vi "Teleop.vi"(10 "Match Info":T1={"Autonomous Elapsed Seconds"=0.0, "TeleOp Elapsed Seconds"=0.0, "Disabled Elapsed Seconds"=0.0, "Visited Autonomous"=FALSE, "Visited TeleOp"=FALSE, "Visited Disabled"=FALSE, "Autonomous Settings"={"Autonomous Style"=enum."Independent", "VI Refnum"=refnum}}, 11 "Call Context":T2) -> ()   [LabVIEW 2012]
doc: "This VI is called for each TeleOp packet received from the DS where the robot is not disabled. It is often used to read from the joysticks and update I/O or to update setpoints for timed control loops. It should complete and return within 20 milliseconds or it may miss DS packets."
uses:
  <vilib>/Rock Robotics/WPI/DriverStation/WPI_DriverStationDerivedRobotMode.ctl
  <vilib>/Rock Robotics/WPI/DriverStation/WPI_DriverStationMatch Info.ctl
  Robot Global Data.vi
  <vilib>/Rock Robotics/WPI/Joystick/WPI_JoystickGetSetRefNum.vi
  <vilib>/Rock Robotics/WPI/RobotDrive/WPI_RobotDriveGetSetRefNum.vi
  Documents/LabVIEW Data/No Wayne Drive/wayne drive.vi
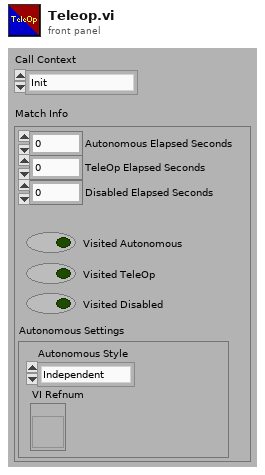
[diagram p1: front panel]
types:
  T1 = typedef "WPI_DriverStationMatch Info.ctl" = cluster{"Autonomous Elapsed Seconds":dbl, "TeleOp Elapsed Seconds":dbl, "Disabled Elapsed Seconds":dbl, "Visited Autonomous":bool, "Visited TeleOp":bool, "Visited Disabled":bool, "Autonomous Settings":cluster{"Autonomous Style":enum16{"Iterative", "Independent"}, "VI Refnum":refnum<vi>}}
  T2 = typedef "WPI_DriverStationDerivedRobotMode.ctl" = enum16{"Init", "Execute", "Stop"}
  T3 = typedef "WPI_JoystickDevRef.ctl" = cluster{"Device":T4}
  T4 = typedef "WPI_JoystickDeviceEnum.ctl" = enum16{"USB 1", "USB 2", "USB 3", "USB 4", "Kinect 1", "Kinect 2"}
  T5 = typedef "WPI_JoystickButtonState.ctl" = cluster{"Button 1":bool, "Button 2":bool, "Button 3":bool, "Button 4":bool, "Button 5":bool, "Button 6":bool, "Button 7":bool, "Button 8":bool, "Button 9":bool, "Button 10":bool, "Button 11":bool, "Button 12":bool}
  T6 = cluster{"axis 1 (x)":dbl, "axis 2 (y)":dbl, "axis 3 (throttle)":dbl, "axis 4":dbl, "axis 5":dbl, "axis 6":dbl}
  T7 = typedef "WPI_RobotDriveDevRef.ctl" = cluster{"DevStatus":errorcluster, "Motors[]":T8[], "Square Inputs":bool, "Max Output":dbl, "Isochronous":bool}
  T8 = typedef "WPI_MotorControlDeviceRef.ctl" = cluster{"DeviceStatus":errorcluster, "Type":enum16{"PWM", "CAN"}, "PWM":cluster{"Digital Module":T9, "PWM Channel":T10, "DeadBand":T11}, "CAN":cluster{"Device Number":u8, "Control Mode":T12, "Semaphore":T13, "Max Vout":dbl}, "Invert":bool, "TransformRef":T14, "InvTransformRef":T14}
  T9 = typedef "FPGA_TypedefDigitalModule.ctl" = enum16{"Digital Module 1", "Digital Module 2"}
  T10 = typedef "FPGA_DIOPWMChannel.ctl" = enum8{"PWM 1", "PWM 2", "PWM 3", "PWM 4", "PWM 5", "PWM 6", "PWM 7", "PWM 8", "PWM 9", "PWM 10", "Invalid"}
  T11 = typedef "WPI_PWMDeadband.ctl" = cluster{"Name":string, "maxPositivePwm":i32, "minPositivePwm":i32, "centerPwm":i32, "maxNegativePwm":i32, "minNegativePwm":i32, "angularRange":u16}
  T12 = typedef "WPI_CANJaguar_ControlMode.ctl" = enum8{"Percent VBus", "Current", "Speed", "Position", "Voltage"}
  T13 = typedef "Semaphore RefNum" = refnum<k1>
  T14 = typedef "WPI_PWMTransform_ConPane.ctl" = refnum<vi>
  T15 = typedef "WPI_RelayDevRef.ctl" = cluster{"DevStatus":errorcluster, "Relay Channel":T16, "Digital Module":T9, "Relay Direction":T17}
  T16 = typedef "FPGA_DIORelayChannel.ctl" = enum8{"Relay 1", "Relay 2", "Relay 3", "Relay 4", "Relay 5", "Relay 6", "Relay 7", "Relay 8", "Invalid"}
  T17 = typedef "WPI_RelayDirection.ctl" = enum16{"Both directions", "Forward only", "Reverse only"}
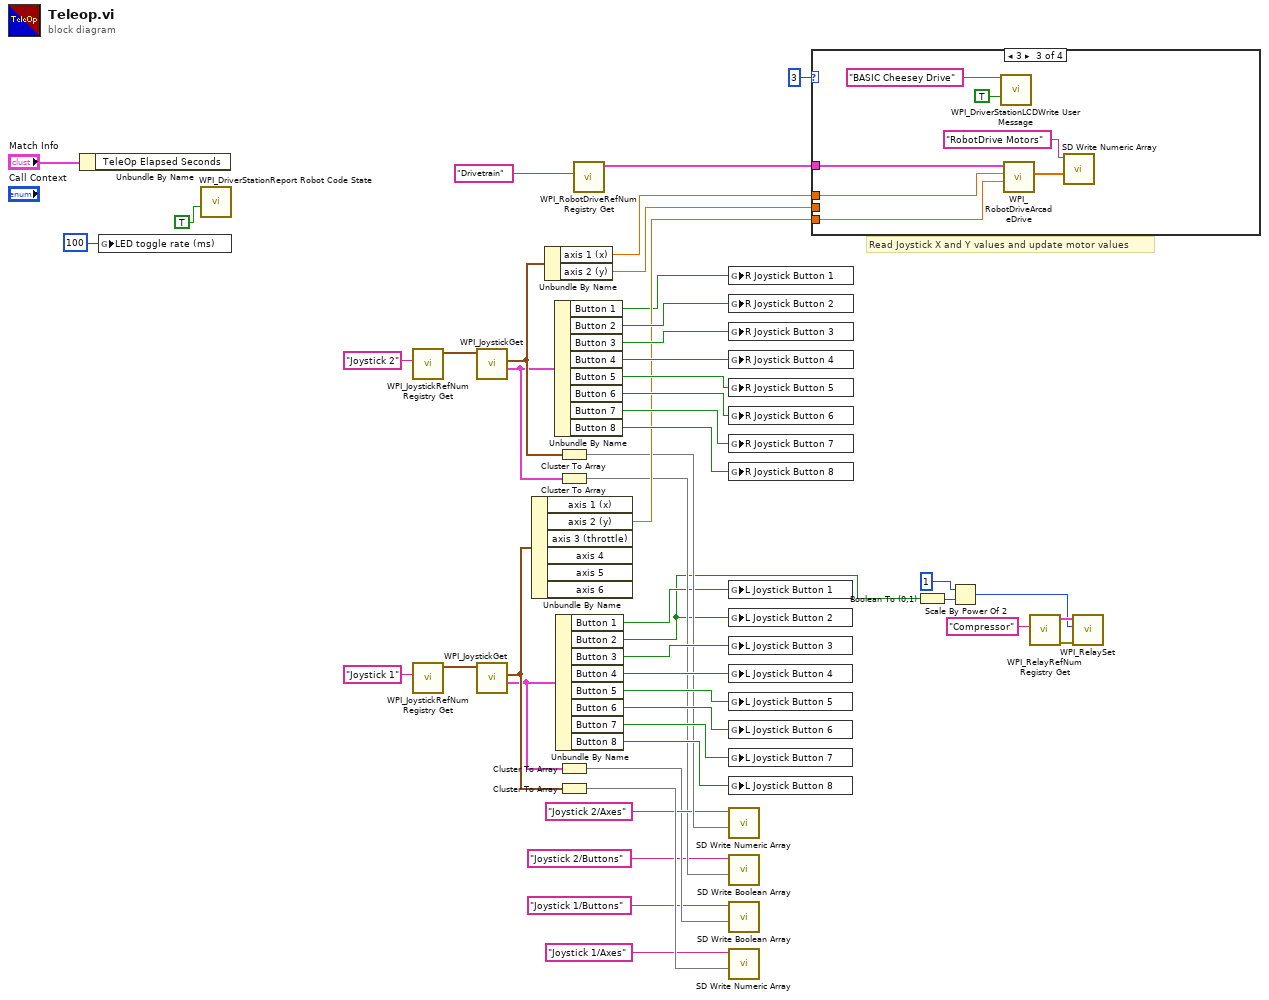
[diagram p0: block diagram]
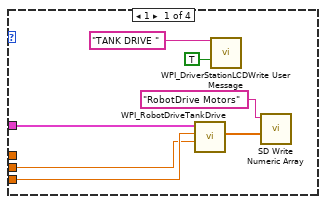
[diagram p2: hidden frame]
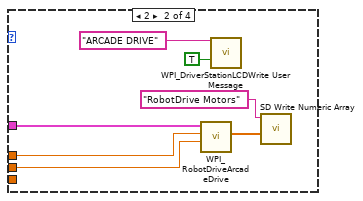
[diagram p3: hidden frame]
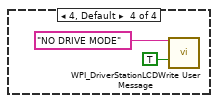
[diagram p4: hidden frame]
diagram:
  # "Read Joystick X and Y values and update motor values"
  n1 = Unbundle By Name("Match Info") -> ()  [unwired: 1 out]
  n2 = global write "Robot Global Data.vi" "LED toggle rate (ms)"(u32 100 ("LED ms toggle rate")) -> ()
  n3 = call <vilib>:"WPI_DriverStationReport Robot Code State.vi"("TeleOp"=TRUE ("Autonomous")) -> ()  [unwired: 10 in, 1 out]
  n4 = call <vilib>:"WPI_JoystickRefNum Registry Get.vi"("refnum name"="Joystick 2") -> ("JoystickDevRef"=w40:T3)  [unwired: 1 in, 9 out]
  n5 = call <vilib>:"WPI_JoystickRefNum Registry Get.vi"("refnum name"="Joystick 1") -> ("JoystickDevRef"=w42:T3)  [unwired: 1 in, 9 out]
  n6 = call <vilib>:"WPI_JoystickGet.vi"("JoystickDevRef"=w40) -> ("Buttons"=w11:T5, "Axes"=w21:T6)  [unwired: 1 in, 4 out]
  n7 = call <vilib>:"WPI_JoystickGet.vi"("JoystickDevRef"=w42) -> ("Buttons"=w14:T5, "Axes"=w19:T6)  [unwired: 1 in, 4 out]
  n8 = Unbundle By Name(w19) -> ("axis 2 (y)"=w23:dbl)  [unwired: 5 out]
  n9 = Unbundle By Name(w21) -> ("axis 1 (x)"=w25:dbl, "axis 2 (y)"=w24:dbl)
  n10 = Unbundle By Name(w11) -> ("Button 1"=w1:bool, "Button 2"=w39:bool, "Button 3"=w38:bool, "Button 4"=w37:bool, "Button 5"=w36:bool, "Button 6"=w35:bool, "Button 7"=w34:bool, "Button 8"=w33:bool)
  n11 = Unbundle By Name(w14) -> ("Button 1"=w9:bool, "Button 2"=w5:bool, "Button 3"=w32:bool, "Button 4"=w31:bool, "Button 5"=w30:bool, "Button 6"=w29:bool, "Button 7"=w28:bool, "Button 8"=w27:bool)
  n12 = Cluster To Array(cluster=w21) -> (array=w22:dbl[])
  n13 = Cluster To Array(cluster=w11) -> (array=w13:bool[])
  n14 = Cluster To Array(cluster=w14) -> (array=w16:bool[])
  n15 = Cluster To Array(cluster=w19) -> (array=w20:dbl[])
  n16 = call <vilib>:"WPI_RobotDriveRefNum Registry Get.vi"("refnum name"="Drivetrain") -> ("RobotDriveDevRef"=w26:T7)  [unwired: 1 in, 9 out]
  n17 = global write "Robot Global Data.vi" "R Joystick Button 1"(w1) -> ()
  n18 = global write "Robot Global Data.vi" "R Joystick Button 2"(w39) -> ()
  n19 = global write "Robot Global Data.vi" "R Joystick Button 3"(w38) -> ()
  n20 = global write "Robot Global Data.vi" "R Joystick Button 4"(w37) -> ()
  n21 = global write "Robot Global Data.vi" "R Joystick Button 5"(w36) -> ()
  n22 = global write "Robot Global Data.vi" "R Joystick Button 6"(w35) -> ()
  n23 = global write "Robot Global Data.vi" "R Joystick Button 7"(w34) -> ()
  n24 = global write "Robot Global Data.vi" "R Joystick Button 8"(w33) -> ()
  n25 = global write "Robot Global Data.vi" "L Joystick Button 1"(w9) -> ()
  n26 = global write "Robot Global Data.vi" "L Joystick Button 2"(w5) -> ()
  n27 = global write "Robot Global Data.vi" "L Joystick Button 3"(w32) -> ()
  n28 = global write "Robot Global Data.vi" "L Joystick Button 4"(w31) -> ()
  n29 = global write "Robot Global Data.vi" "L Joystick Button 5"(w30) -> ()
  n30 = global write "Robot Global Data.vi" "L Joystick Button 6"(w29) -> ()
  n31 = global write "Robot Global Data.vi" "L Joystick Button 7"(w28) -> ()
  n32 = global write "Robot Global Data.vi" "L Joystick Button 8"(w27) -> ()
  n33 = call <vilib>:"SD Write Numeric Array.vi"("Numeric Array"=w22, "Name"="Joystick 2/Axes") -> ()  [unwired: 8 in, 2 out]
  n34 = call <vilib>:"SD Write Boolean Array.vi"("Boolean Array"=w13, "Name"="Joystick 2/Buttons") -> ()  [unwired: 8 in, 2 out]
  n35 = call <vilib>:"SD Write Boolean Array.vi"("Boolean Array"=w16, "Name"="Joystick 1/Buttons") -> ()  [unwired: 8 in, 2 out]
  n36 = call <vilib>:"SD Write Numeric Array.vi"("Numeric Array"=w20, "Name"="Joystick 1/Axes") -> ()  [unwired: 8 in, 2 out]
  n37 = case shown="3" 3 {
    tunnel: w26 -> [w52 w58 w67 _]
    tunnel: w25 -> [_ w57 w66 _]
    tunnel: w24 -> [w48 w56 _ _]
    tunnel: w23 -> [w49 _ w62 _]
    frame 1 {
      n38 = call <vilib>:"WPI_RobotDriveTankDrive.vi"("Right axis value"=w48, "Left axis value"=w49, "RobotDriveDevRef"=w52) -> ("Motor Values"=w50:dbl[])  [unwired: 6 in, 2 out]
      n39 = call <vilib>:"WPI_DriverStationLCDWrite User Message.vi"("line text"="TANK DRIVE ", "clear line before write (T)"=TRUE) -> ()  [unwired: 13 in, 1 out]
      n40 = call <vilib>:"SD Write Numeric Array.vi"("Numeric Array"=w50, "Name"="RobotDrive Motors") -> ()  [unwired: 8 in, 2 out]
    }
    frame 2 {
      n41 = call-poly <vilib>:"WPI_RobotDriveArcadeDrive.vi"("Y axis value"=w56, "X axis value"=w57, "RobotDriveDevRef"=w58) -> ("Motor Values"=w55:dbl[])  [unwired: 6 in, 2 out]
      n42 = call <vilib>:"WPI_DriverStationLCDWrite User Message.vi"("line text"="ARCADE DRIVE", "clear line before write (T)"=TRUE) -> ()  [unwired: 13 in, 1 out]
      n43 = call <vilib>:"SD Write Numeric Array.vi"("Numeric Array"=w55, "Name"="RobotDrive Motors") -> ()  [unwired: 8 in, 2 out]
    }
    frame 3 {
      n44 = call <vilib>:"WPI_DriverStationLCDWrite User Message.vi"("line text"="BASIC Cheesey Drive", "clear line before write (T)"=TRUE) -> ()  [unwired: 13 in, 1 out]
      n45 = call-poly <vilib>:"WPI_RobotDriveArcadeDrive.vi"("Y axis value"=w62, "X axis value"=w66, "RobotDriveDevRef"=w67) -> ("Motor Values"=w65:dbl[])  [unwired: 6 in, 2 out]
      n46 = call <vilib>:"SD Write Numeric Array.vi"("Numeric Array"=w65, "Name"="RobotDrive Motors") -> ()  [unwired: 8 in, 2 out]
    }
    frame 4, Default {
      n47 = call <vilib>:"WPI_DriverStationLCDWrite User Message.vi"("line text"="NO DRIVE MODE", "clear line before write (T)"=TRUE) -> ()  [unwired: 13 in, 1 out]
    }
  }
  n48 = Boolean To (0,1)(Boolean=w5) -> (0, 1=w3:i16)
  n49 = Scale By Power Of 2(n=i16 1, x=w3) -> (x*2^n=w2:i16)
  n50 = call <vilib>:"WPI_RelayRefNum Registry Get.vi"("refnum name"="Compressor") -> ("error out"=w7:errorcluster, "RelayDevRef"=w8:T15)  [unwired: 9 in]
  n51 = call <vilib>:"WPI_RelaySet.vi"("error in (no error)"=w7, "RelayValue"=w2, "RelayDevRef"=w8) -> ()  [unwired: 7 in, 2 out]
